vi "全局变量.vi"() -> ()   [LabVIEW 2018]
panel:
  out "error out":errorcluster caption="错误输出"
  out "总帧数":dbl
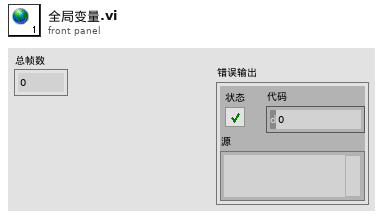
[diagram p1: front panel]
diagram:
